vi "PH_CheckErrorCode.vi"(0 "errcode":i32, 11 "error in (no error)":errorcluster) -> (4 "Is Error":bool, 15 "error out":errorcluster)   [LabVIEW 8.6]
uses:
  MT Scan/SubVIs/PHLib.dll
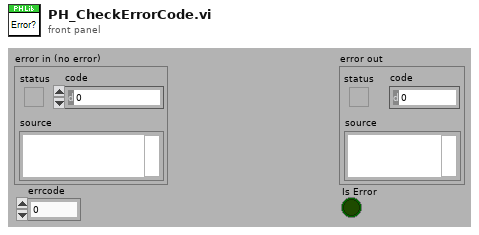
[diagram p1: front panel]
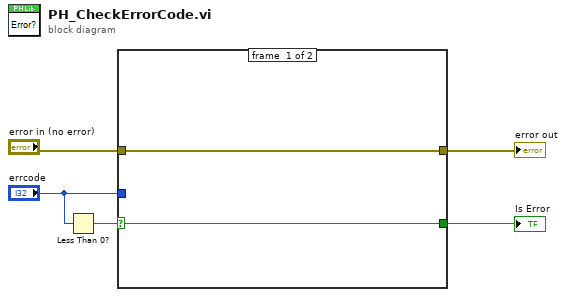
[diagram p0: block diagram]
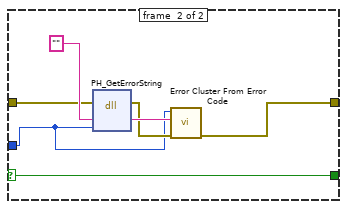
[diagram p2: hidden frame]
diagram:
  n1 = Less Than 0?(x="errcode") -> (x < 0?=w3:bool)
  n2 = case shown="True" w3 {
    selector: w3 -> [w6 w8]
    tunnel: "error in (no error)" -> [w7 w11]
    tunnel: "errcode" -> [_ w10]
    tunnel: [w7 w9] -> w2
    tunnel: [w6 w8] -> w1
    frame #0 {
    }
    frame #1 {
      n3 = dll-call lib="C:/LabVIEW Programs/MT Scan/SubVIs/PHLib.dll" fn="PH_GetErrorString"(error in=w11, "errstring"="", "errcode"=w10) -> (error out=w13:errorcluster, "errstring"=w14:string)  [unwired: 4 in, 1 out]
      n4 = call <vilib>:"Error Cluster From Error Code.vi"("error in (no error)"=w13, "error message (\"\")"=w14, "error code (0)"=w10) -> ("error out"=w9:errorcluster)  [unwired: 6 in]
    }
  }
  "error out" <- w2
  "Is Error" <- w1
